vi "copy exif tags.vi"(8 "error in":errorcluster, 10 "destination":path, 11 "source":path) -> (0 "error out":errorcluster, 1 "standard error":string)   [LabVIEW 2023]
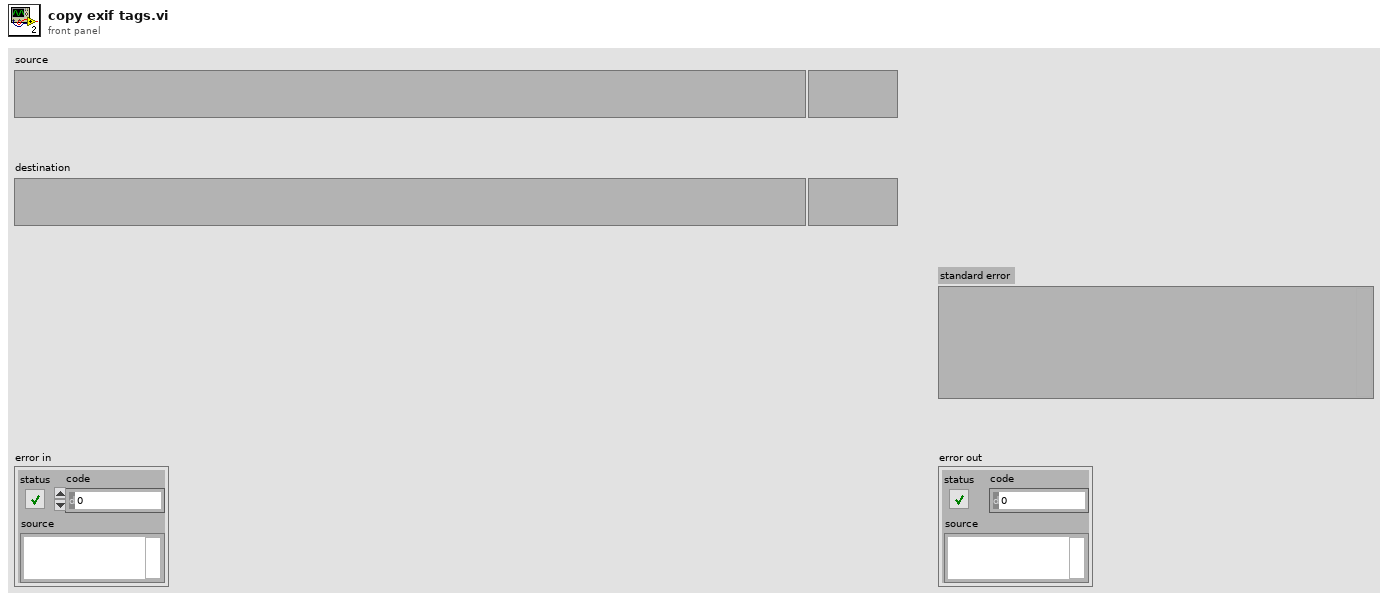
[diagram p1: front panel]
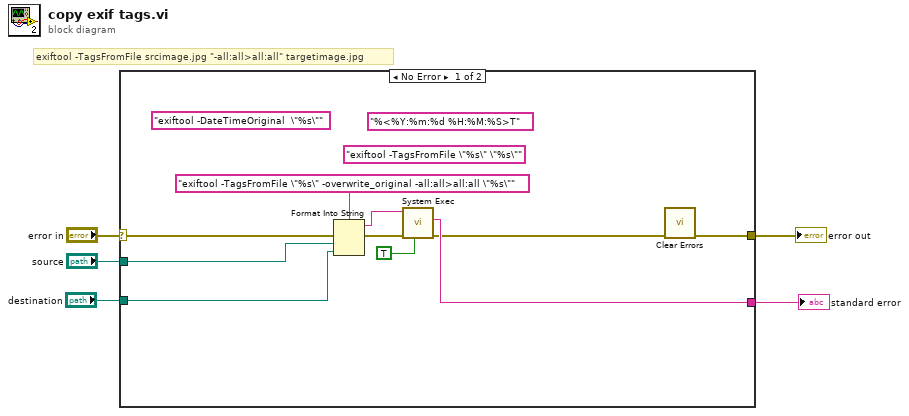
[diagram p0: block diagram]
diagram:
  # "exiftool -TagsFromFile srcimage.jpg \"-all:all>all:all\" targetimage.jpg"
  n1 = case shown="No Error" "error in" {
    selector: "error in" -> [w10 w16]
    tunnel: "source" -> [w14 _]
    tunnel: [w8 w16] -> w4
    tunnel: [w9 _] -> w2
    tunnel: "destination" -> [w6 _]
    frame No Error {
      (unwired) "exiftool -TagsFromFile \"%s\" \"%s\"" ("command line")
      (unwired) "exiftool -DateTimeOriginal  \"%s\"" ("command line")
      (unwired) "%<%Y:%m:%d %H:%M:%S>T" ("format string")
      n2 = Format Into String(format string="exiftool -TagsFromFile \"%s\" -overwrite_original -all:all>all:all \"%s\"" ("command line"), error in=w10, w14, w6) -> (resulting string=w12:string, error out=w11:errorcluster)  [unwired: 1 in]
      n3 = call <vilib>:"System Exec.vi"("run minimized? (F)"=TRUE, "error in (no error)"=w11, "command line"=w12) -> ("error out"=w7:errorcluster, "standard error"=w9:string)  [unwired: 5 in, 2 out]
      n4 = call <vilib>:"Clear Errors.vi"("error in (no error)"=w7) -> ("error out"=w8:errorcluster)  [unwired: 5 in, 1 out]
    }
    frame Error {
    }
  }
  "error out" <- w4
  "standard error" <- w2
